vi "Graphics-LTRB to LTWH (clusters).vi"(4 "LTRB":T2) -> (1 "LTWH":T1)   [LabVIEW 2020]
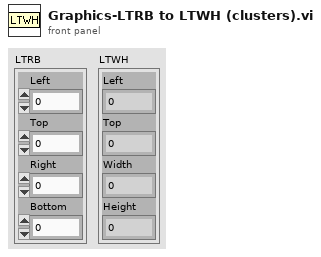
[diagram p1: front panel]
types:
  T1 = cluster{"Left":i16, "Top":i16, "Width":i16, "Height":i16}
  T2 = cluster{"Left":i16, "Top":i16, "Right":i16, "Bottom":i16}
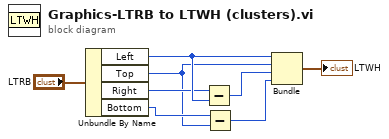
[diagram p0: block diagram]
diagram:
  n1 = Unbundle By Name("LTRB") -> ("Left"=w5:i16, "Top"=w2:i16, "Right"=w4:i16, "Bottom"=w3:i16)
  n2 = Subtract(x=w4, y=w5) -> (x-y=w8:i16)
  n3 = Subtract(x=w3, y=w2) -> (x-y=w7:i16)
  n4 = Bundle("Left"=w5, "Top"=w2, w8, w7) -> (→"LTWH":cluster{"Left":i16, "Top":i16, i16, i16})  [unwired: 1 in]
